vi "vendingmachine.vi"() -> ()   [LabVIEW 2020]
uses:
  Control 3.ctl
panel:
  in  "stop":bool
  out "Message to User":string
  out "Change Returned":dbl format="%.2f"
  in  "Pepsi":bool
  in  "Coke":bool
  out "Coke Display":u16(ring)
  in  "Return Change":bool
  out "Value Deposited":dbl format="%.2f"
  in  "Dime":bool
  in  "Nickel":bool
  in  "Quarter":bool
  # "$0.75"
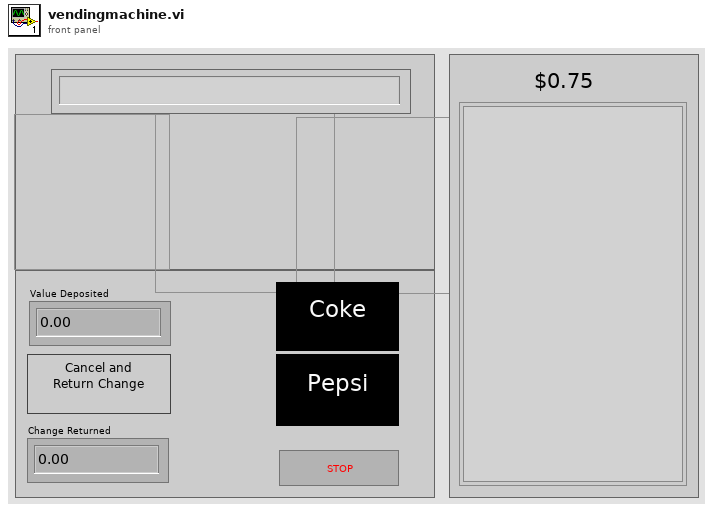
[diagram p1: front panel]
types:
  T1 = typedef "Control 3.ctl" = enum16{"Initialize", "Stop", "Wait for gui event", "Vend and return change", "Cancel and return change"}
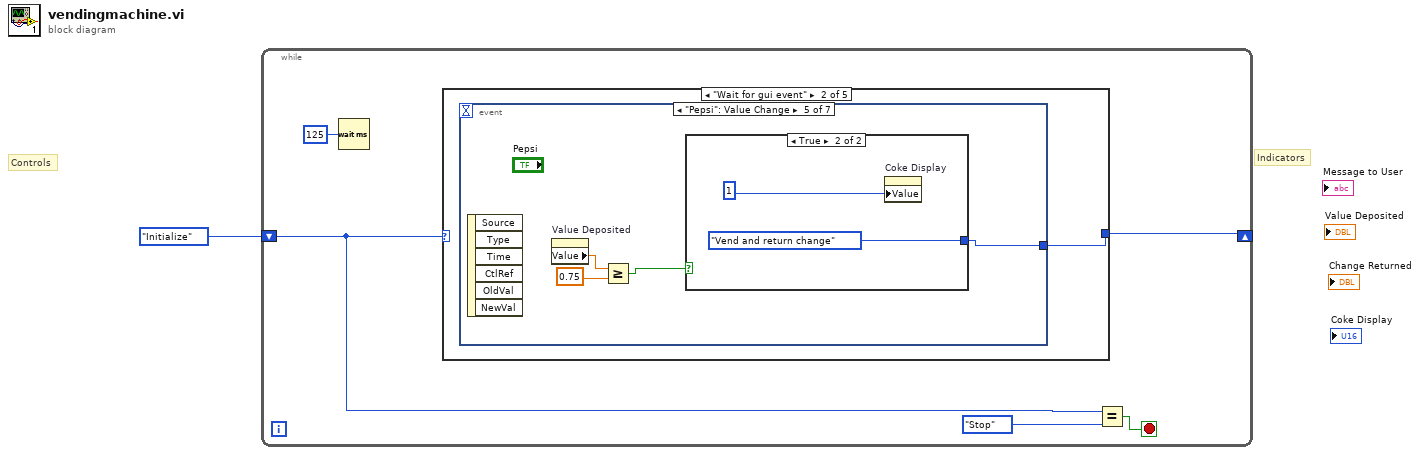
[diagram p0: block diagram]
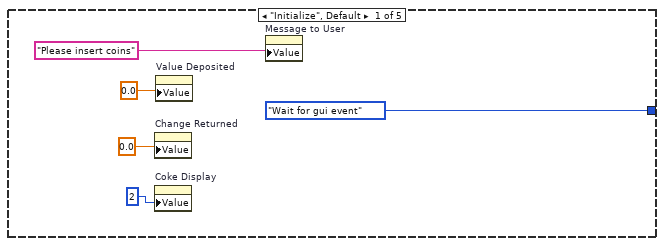
[diagram p2: hidden frame]
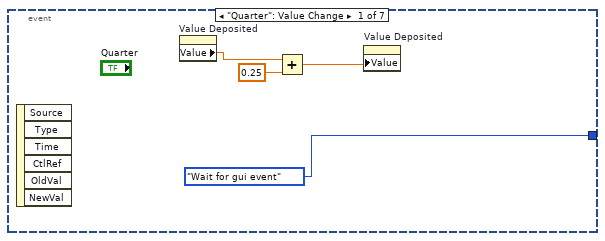
[diagram p3: hidden frame]
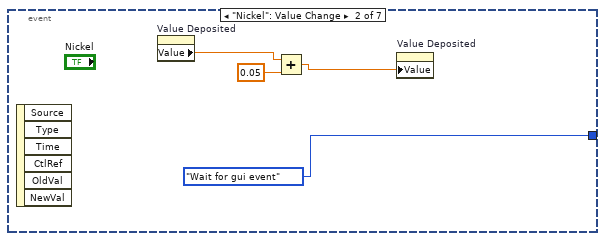
[diagram p4: hidden frame]
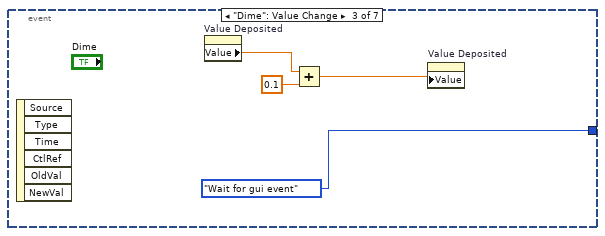
[diagram p5: hidden frame]
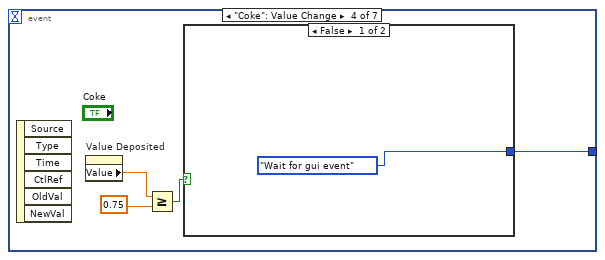
[diagram p6: hidden frame]
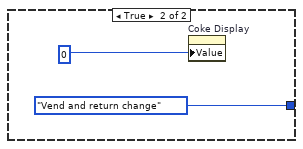
[diagram p7: hidden frame]
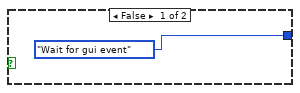
[diagram p8: hidden frame]
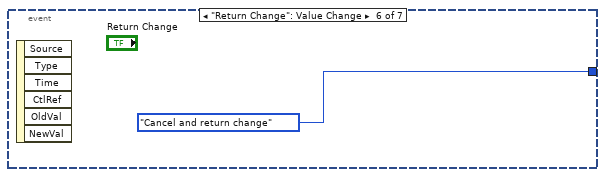
[diagram p9: hidden frame]
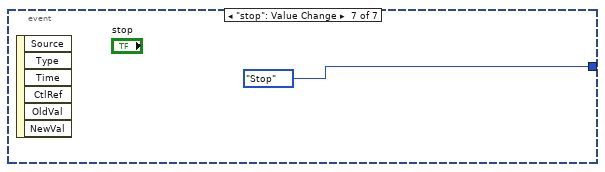
[diagram p10: hidden frame]
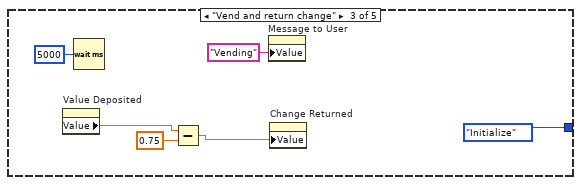
[diagram p11: hidden frame]
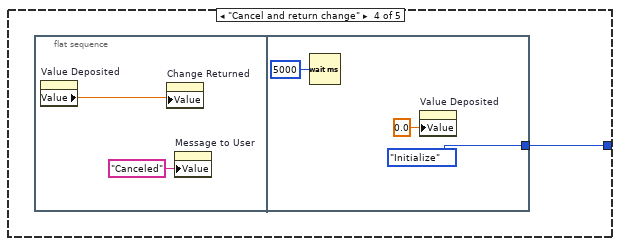
[diagram p12: hidden frame]
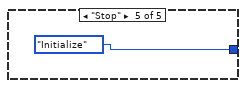
[diagram p13: hidden frame]
diagram:
  # "Indicators"
  # "Controls"
  n1 = while {
    shift-right: [w2] -> _
    shift-left: Control_3."Initialize" -> [w4]
    stop <- w6 stop-if-true
    n2 = Wait (ms)(milliseconds to wait=u32 125) -> ()  [unwired: 1 out]
    n3 = case shown="\"Wait for gui event\"" w4 {
      tunnel: [Control_3."Wait for gui event" w12 Control_3."Initialize" w47 Control_3."Initialize"] -> w2
      frame "Initialize", Default {
        n4 = property on="Change Returned" class="DigNum (strict)"("Value"=0.0 ("Change Returned")) -> ()  [unwired: 2 in, 2 out]
        n5 = property on="Coke Display" class="Ring (strict)"("Value"=u16 2 ("Coke Display")) -> ()  [unwired: 2 in, 2 out]
        n6 = property on="Value Deposited" class="DigNum (strict)"("Value"=0.0 ("Value Deposited")) -> ()  [unwired: 2 in, 2 out]
        n7 = property on="Message to User" class="Str"("Value"="Please insert coins" ("Message to User")) -> ()  [unwired: 2 in, 2 out]
      }
      frame "Wait for gui event" {
        n8 = event shown="[4] \"Pepsi\": Value Change" {
          selector: _ -> [_ _ _ _ _ _ _]
          dyn-events: _ -> [_ _ _ _ _ _ _]
          timeout: _ -> [_ _ _ _ _ _ _]
          tunnel: [Control_3."Wait for gui event" Control_3."Wait for gui event" Control_3."Wait for gui event" w28 w32 Control_3."Cancel and return change" Control_3."Stop"] -> w12
          event "Quarter": Value Change {
            n9 = event-data() -> ()  [unwired: 1 in, 6 out]
            n10 = property on="Value Deposited" class="DigNum (strict)"() -> ("Value"=w14:dbl)  [unwired: 2 in, 2 out]
            n11 = Add(x=w14, y=0.25) -> (x+y=w15:dbl)
            n12 = property on="Value Deposited" class="DigNum (strict)"("Value"=w15) -> ()  [unwired: 2 in, 2 out]
          }
          event "Nickel": Value Change {
            n13 = event-data() -> ()  [unwired: 1 in, 6 out]
            n14 = property on="Value Deposited" class="DigNum (strict)"() -> ("Value"=w18:dbl)  [unwired: 2 in, 2 out]
            n15 = Add(x=w18, y=0.05) -> (x+y=w17:dbl)
            n16 = property on="Value Deposited" class="DigNum (strict)"("Value"=w17) -> ()  [unwired: 2 in, 2 out]
          }
          event "Dime": Value Change {
            n17 = event-data() -> ()  [unwired: 1 in, 6 out]
            n18 = property on="Value Deposited" class="DigNum (strict)"() -> ("Value"=w22:dbl)  [unwired: 2 in, 2 out]
            n19 = Add(x=w22, y=0.1) -> (x+y=w21:dbl)
            n20 = property on="Value Deposited" class="DigNum (strict)"("Value"=w21) -> ()  [unwired: 2 in, 2 out]
          }
          event "Coke": Value Change {
            n21 = event-data() -> ()  [unwired: 1 in, 6 out]
            n22 = property on="Value Deposited" class="DigNum (strict)"() -> ("Value"=w26:dbl)  [unwired: 2 in, 2 out]
            n23 = Greater Or Equal?(x=w26, y=0.75) -> (x >= y?=w27:bool)
            n24 = case shown="False" w27 {
              tunnel: [Control_3."Wait for gui event" Control_3."Vend and return change"] -> w28
              frame False {
              }
              frame True {
                n25 = property on="Coke Display" class="Ring (strict)"("Value"=u16 0 ("Coke Display")) -> ()  [unwired: 2 in, 2 out]
              }
            }
          }
          event "Pepsi": Value Change {
            n26 = event-data() -> ()  [unwired: 1 in, 6 out]
            n27 = property on="Value Deposited" class="DigNum (strict)"() -> ("Value"=w33:dbl)  [unwired: 2 in, 2 out]
            n28 = Greater Or Equal?(x=w33, y=0.75) -> (x >= y?=w34:bool)
            n29 = case shown="True" w34 {
              tunnel: [Control_3."Wait for gui event" Control_3."Vend and return change"] -> w32
              frame False {
              }
              frame True {
                n30 = property on="Coke Display" class="Ring (strict)"("Value"=u16 1 ("Coke Display")) -> ()  [unwired: 2 in, 2 out]
              }
            }
          }
          event "Return Change": Value Change {
            n31 = event-data() -> ()  [unwired: 1 in, 6 out]
          }
          event "stop": Value Change {
            n32 = event-data() -> ()  [unwired: 1 in, 6 out]
          }
        }
      }
      frame "Vend and return change" {
        n33 = property on="Value Deposited" class="DigNum (strict)"() -> ("Value"=w42:dbl)  [unwired: 2 in, 2 out]
        n34 = Wait (ms)(milliseconds to wait=u32 5000) -> ()  [unwired: 1 out]
        n35 = Subtract(x=w42, y=0.75) -> (x-y=w41:dbl)
        n36 = property on="Message to User" class="Str"("Value"="Vending" ("Message to User")) -> ()  [unwired: 2 in, 2 out]
        n37 = property on="Change Returned" class="DigNum (strict)"("Value"=w41) -> ()  [unwired: 2 in, 2 out]
      }
      frame "Cancel and return change" {
        n38 = flat-sequence {
          tunnel: [Control_3."Initialize"] -> w47
          frame #0 {
            n39 = property on="Value Deposited" class="DigNum (strict)"() -> ("Value"=w49:dbl)  [unwired: 2 in, 2 out]
            n40 = property on="Change Returned" class="DigNum (strict)"("Value"=w49) -> ()  [unwired: 2 in, 2 out]
            n41 = property on="Message to User" class="Str"("Value"="Canceled" ("Message to User")) -> ()  [unwired: 2 in, 2 out]
          }
          frame #1 {
            n42 = Wait (ms)(milliseconds to wait=u32 5000) -> ()  [unwired: 1 out]
            n43 = property on="Value Deposited" class="DigNum (strict)"("Value"=0.0 ("Value Deposited")) -> ()  [unwired: 2 in, 2 out]
          }
        }
      }
      frame "Stop" {
      }
    }
    n44 = Equal?(x=w4, y=Control_3."Stop") -> (x = y?=w6:bool)
  }
